vi "Check error.vi"(8 "error in (no error)":errorcluster, 11 "AlphaStep One in":refnum<class "AlphaStep One.lvclass">) -> (0 "error out":errorcluster, 2 "Error code":i32, 3 "AlphaStep One out":refnum<class "AlphaStep One.lvclass">)   [LabVIEW 2015, in "AlphaStep One.lvclass"]
uses:
  AlphaStep One.lvclass
  AlphaStep One.lvclass/AlphaStep One.ctl
  Serial Device/Serial Device.lvclass
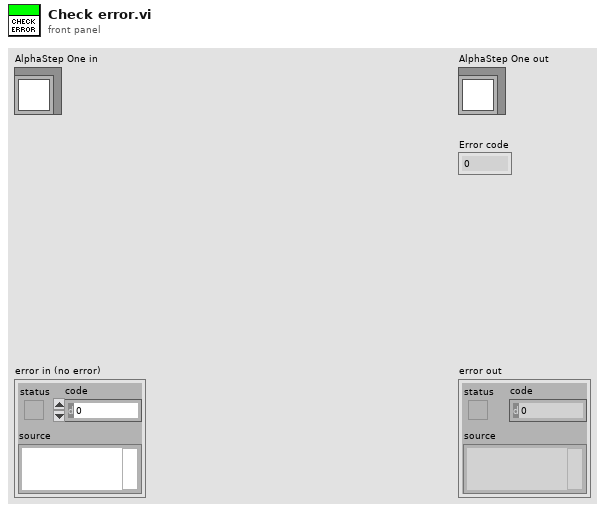
[diagram p1: front panel]
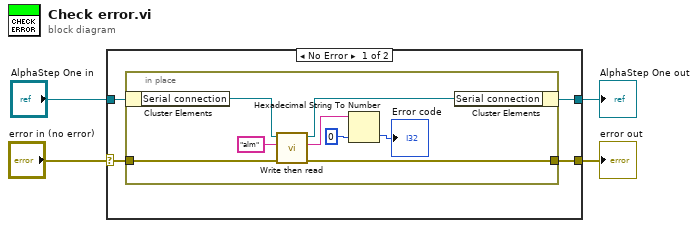
[diagram p0: block diagram]
diagram:
  n1 = case shown="No Error" "error in (no error)" {
    selector: "error in (no error)" -> [w6 w18]
    tunnel: [w5 w18] -> w3
    tunnel: "AlphaStep One in" -> [w8 w17]
    tunnel: [w7 w17] -> w1
    frame No Error {
      n2 = in-place {
        in-place-border: w6 -> [w10]
        in-place-border: [w9] -> w5
        n3 = in-place-cluster #1(w8) -> ("Serial connection"=w16:refnum<class "Serial Device.lvclass">)
        n4 = call "Write then read.vi"("error in (no error)"=w10, "TX Data"="alm", "Serial Device in"=w16) -> ("error out"=w9:errorcluster, "RX Data"=w14:string, "Serial Device out"=w11:refnum<class "Serial Device.lvclass">)  [unwired: 6 in]
        n5 = Hexadecimal String To Number(string=w14, default (0uL)=0 ("default (0 U32)")) -> (number=→"Error code":i32)  [unwired: 1 in, 1 out]
        n6 = in-place-cluster #1("Serial connection"=w11) -> (w7:refnum<class "AlphaStep One.lvclass">)
      }
    }
    frame Error {
    }
  }
  "error out" <- w3
  "AlphaStep One out" <- w1
